vi "Get Active Scale.vi"(7 "error in (no error)":errorcluster, 10 "references":T1) -> (0 "error out":errorcluster, 2 "Index":i32, 3 "references out":T1)   [LabVIEW 2013, in "Scaling editor node.lvclass"]
uses:
  Scaling editor node.lvclass
  <vilib>/NI/DCAF Table API/Table Manager/object ref.ctl
  <vilib>/NI/Tag Bus Data Framework/Configuration Editor/Classes/Engine Parent/Engine Parent Editor Node.lvclass
  <vilib>/NI/Tag Bus Data Framework/Configuration Editor/Classes/Module editor node/module editor node.lvclass
  Scaling editor node.lvclass/Scaling editor node.ctl
  accessors/Read active scale index .vi
  <vilib>/NI/DCAF Table API/Table Manager/Table Manager.lvclass
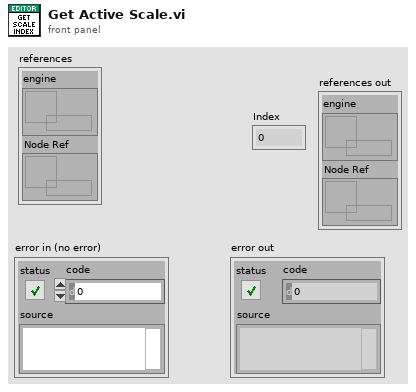
[diagram p1: front panel]
types:
  T1 = typedef "Table Manager.lvlib/Table Manager.lvclass/object ref.ctl" = cluster{"engine":refnum<data-value>, "Node Ref":refnum<data-value>}
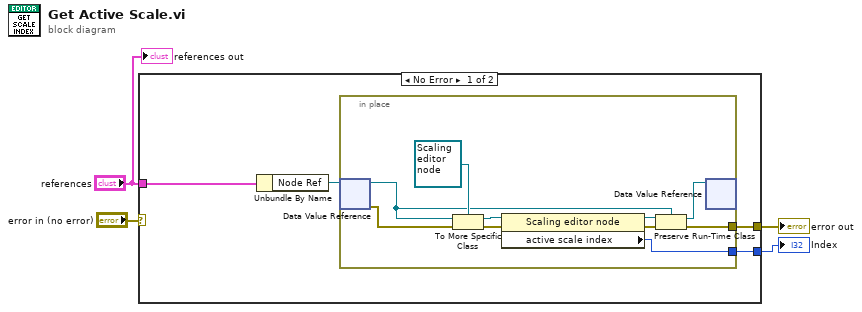
[diagram p0: block diagram]
diagram:
  n1 = case shown="No Error" "error in (no error)" {
    selector: "error in (no error)" -> [_ w19]
    tunnel: [w8 w19] -> w3
    tunnel: [w6 _] -> w2
    tunnel: "references" -> [w5 _]
    frame No Error {
      n2 = Unbundle By Name(w5) -> ("Node Ref"=w7:refnum<data-value>)
      n3 = in-place {
        in-place-border: [w13] -> w8
        in-place-border: [w9] -> w6
        n4 = in-place-dvr #1(w7) -> (w11:refnum<class "module editor node.lvclass">, w16:errorcluster)
        n5 = To More Specific Class(target class=refnum<class "Scaling editor node.lvclass"> refnum ("Scaling editor node"), reference=w11, error in=w16) -> (specific class reference=w18:refnum<class "Scaling editor node.lvclass">, error out=w17:errorcluster)
        n6 = property class="Scaling editor node"(reference=w18, error in=w17) -> (reference out=w12:refnum<class "Scaling editor node.lvclass">, error out=w14:errorcluster, "active scale index "=w9:i32)
        n7 = Preserve Run-Time Class(object in=w12, error in=w14, 2:w11) -> (object out=w10:refnum<class "module editor node.lvclass">, error out=w13:errorcluster)
        n8 = in-place-dvr #1(w10) -> ()  [unwired: 2 out]
      }
    }
    frame Error {
    }
  }
  "Index" <- w2
  "error out" <- w3
  "references out" <- "references"
